vi "HMI.vi"(8 "error in (no error)":errorcluster caption="entrée d'erreur (pas d'erreur)", 11 "Class Popup Autotest (Default) en entrée":refnum<class "Popup Autotest_Without_Actor.lvclass">) -> (0 "error out":errorcluster caption="sortie d'erreur", 1 "Input":string, 2 "Autotest":bool, 3 "Class Popup Autotest (Default) en sortie":refnum<class "Popup Autotest_Without_Actor.lvclass">)   [LabVIEW 2020, in "Library Instrument & Equipement.lvlib" / "Library Popup.lvlib" / "Popup Autotest_Without_Actor.lvclass"]
uses:
  Popup Autotest_Without_Actor.lvclass
  C:/Users/ngarcin/OneDrive - Altyor/Standard TB/Class/Popup/Class Popup (Main)/Class Popup (Main).lvclass
  C:/Users/ngarcin/OneDrive - Altyor/Standard TB/Class/Popup/Class Popup Autotest (Default)/Popup Autotest (Default).lvclass
  Commun VI/TypeDef/Commande Popup autotest/Commande element autotest.ctl
  Variable Instr.vi
  Instrument/Instrument (Default)/Class Instrument (Default).lvclass
  Class Popup Autotest (Default)/Popup Autotest (Default).lvclass
  Popup Autotest_Without_Actor.lvclass/Popup Autotest_Without_Actor.ctl
panel:
  out "Element test":T2
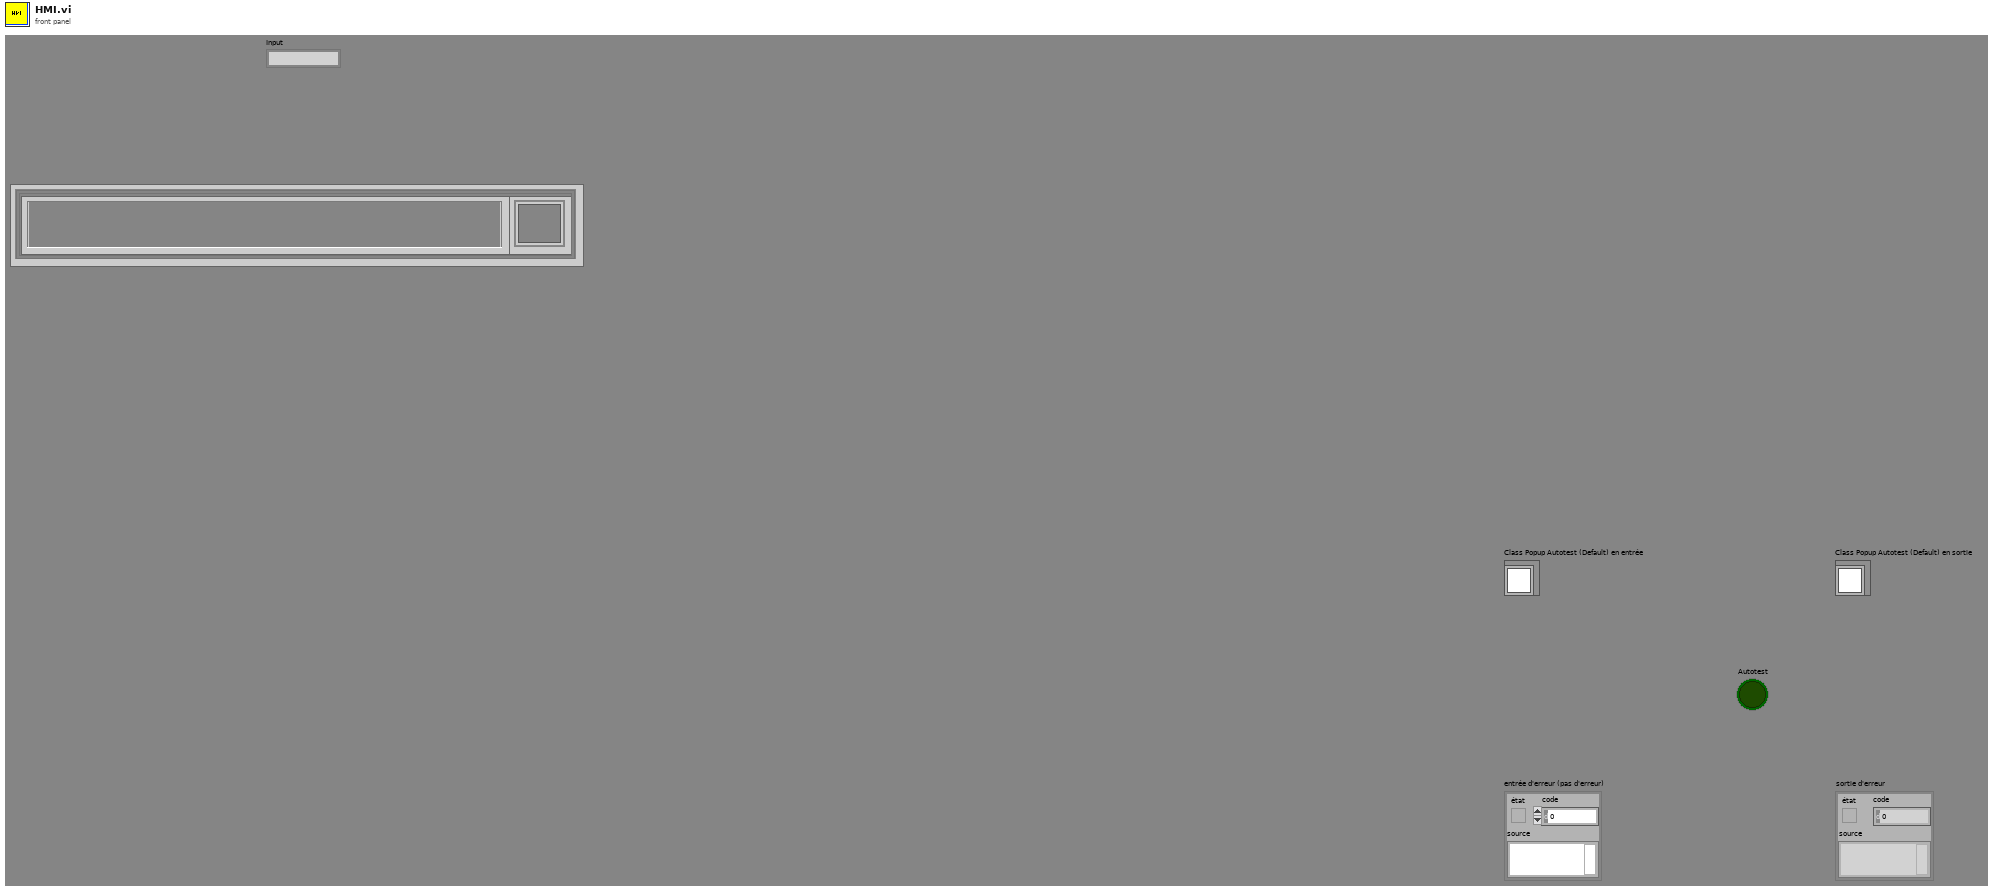
[diagram p1: front panel]
types:
  T1 = typedef "Commande element autotest.ctl" = cluster{"Instrument":string, "Etat":cluster{"Menu déroulant":u16}}
  T2 = cluster{"Element autotest":T1, "Element autotest 2":T1, "Element autotest 3":T1, "Element autotest 4":T1, "Element autotest 5":T1, "Element autotest 6":T1, "Element autotest 7":T1, "Element autotest 8":T1, "Element autotest 9":T1}
  T3 = cluster{"Name":string, "Instrument":refnum<class "Class Instrument (Default).lvclass">, "Close After Autotest":bool}[]
  T4 = cluster{"Name":string, "Instrument":refnum<class "Class Instrument (Default).lvclass">, "Close After Autotest":bool}
  T5 = typedef "LVRectTypeDef.ctl" = cluster{"Left":i16, "Top":i16, "Right":i16, "Bottom":i16}
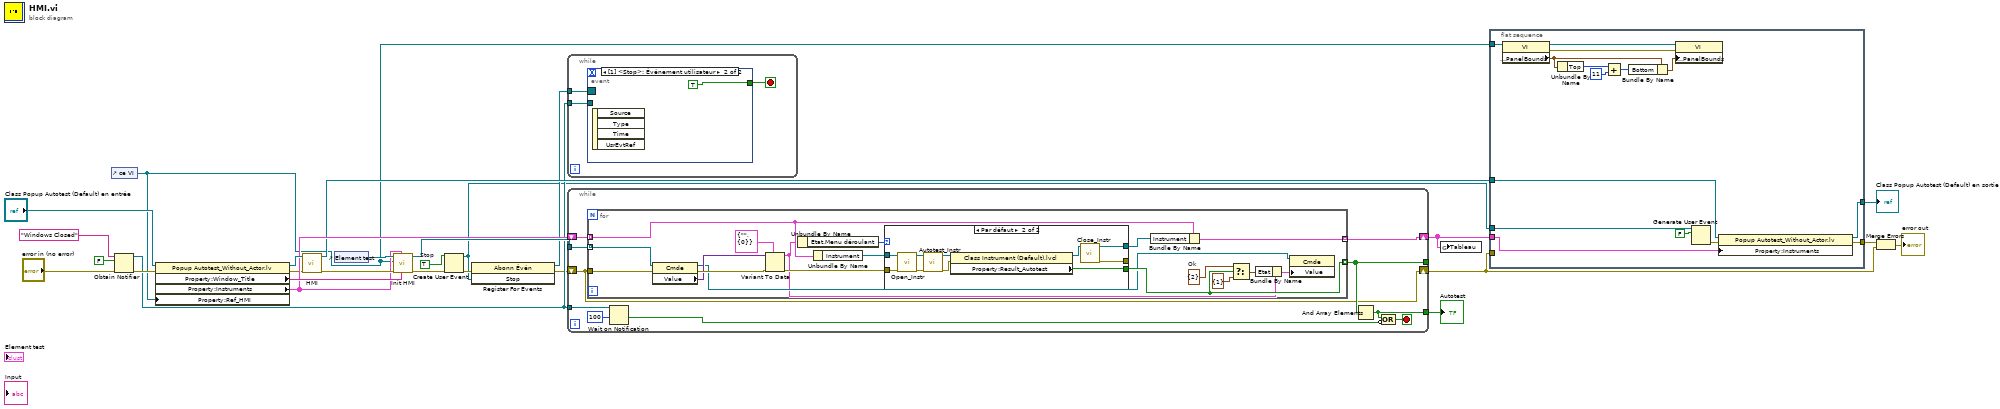
[diagram p0: block diagram]
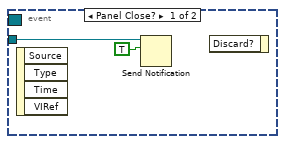
[diagram p2: hidden frame]
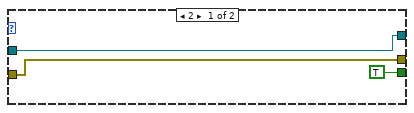
[diagram p3: hidden frame]
diagram:
  w12 = TRUE  # Stop
  n1 = control-ref of="ce VI"() -> (w1:refnum<vi>)
  n2 = Obtain Notifier(name (unnamed)="Windows Closed" ("nom (aucun)"), notification data type=FALSE, error in (no error)="error in (no error)") -> (notifier out=w14:refnum<notifier>, error out=w17:errorcluster)  [unwired: 1 in, 1 out]
  n3 = property class="Popup Autotest_Without_Actor.lv"(reference="Class Popup Autotest (Default) en entrée", error in=w17, "Property:Ref_HMI"=w1) -> (reference out=w27:refnum<class "Popup Autotest_Without_Actor.lvclass">, error out=w2:errorcluster, "Property:Window_Title"=w24:string, "Property:Instruments"=w21:T3)
  n4 = call-parent "HMI.vi"("error in (no error)"=w2, "Class Popup Autotest (Default) en entrée"=w27) -> ("error out"=w23:errorcluster, "Class Popup Autotest (Default) en sortie"=w18:refnum<class "Popup Autotest_Without_Actor.lvclass">)  [unwired: 6 in, 2 out]
  n5 = control-ref of="Element test"() -> (w25:refnum<vi>)
  n6 = call "Init HMI.vi"("Window_Title"=w24, "Instruments"=w21, "entrée d'erreur (pas d'erreur)"=w23, "ce VI"=w1, "Cluster en entrée"=w25) -> ("sortie d'erreur"=w11:errorcluster, "Ref Cmd Cluster element"=w22:refnum<vi>[])  [unwired: 5 in]
  n7 = Create User Event(user event datatype=w12, error in=w11) -> (user event=w8:refnum<user-event>, error out=w10:errorcluster)
  n8 = register-events(error in=w10, w8) -> (reference out=w13:refnum<event-registration>, error out=w9:errorcluster)  [unwired: 1 in]
  n9 = while {
    tunnel: w14 -> [w30]
    tunnel: w13 -> [w29]
    stop <- w28 stop-if-true
    n10 = event shown="[1] <Stop>: Événement utilisateur" {
      selector: w29 -> [_ _]
      dyn-events: _ -> [_ _]
      timeout: _ -> [_ _]
      tunnel: w30 -> [w32 _]
      tunnel: [_ TRUE] -> w28
      event Panel Close? {
        n11 = event-data() -> ()  [unwired: 1 in, 4 out]
        n12 = Send Notification(notification=TRUE, notifier=w32) -> ()  [unwired: 1 in, 2 out]
        n13 = event-data() -> ()  [unwired: 2 in, 1 out]
      }
      event User Event {
        n14 = event-data() -> ()  [unwired: 1 in, 4 out]
      }
    }
  }
  n15 = while {
    tunnel: [w38] -> _
    tunnel: w22 -> [w43]
    shift-right: [w34] -> w4
    shift-left: w9 -> [w34]
    shift-right: [w41] -> w3
    shift-left: w21 -> [w42]
    tunnel: w14 -> [w40]
    tunnel: [w37] -> w7
    stop <- w35 stop-if-true
    n16 = for {
      tunnel: w42 -> [w61] mode=indexing
      tunnel: [w60] -> w41 mode=indexing
      tunnel: [w55] -> w38 mode=indexing
      tunnel: w43 -> [w57] mode=indexing
      tunnel: w34 -> [w44]
      w56 = cluster{"Menu déroulant":u16} {"Menu déroulant"=2}  # Ok
      n17 = property class="Cmde"(reference=w57, error in=w44) -> (reference out=w51:refnum<vi>, error out=w58:errorcluster, "Value"=w53:variant)
      n18 = Variant To Data(error in=w58, type=T1 {"Instrument"="", "Etat"={"Menu déroulant"=0}} ("Element autotest"), Variant=w53) -> (data=w46:T1, error out=w48:errorcluster)
      n19 = Unbundle By Name(w46) -> ("Etat.Menu déroulant"=w45:u16)
      n20 = Unbundle By Name(w61) -> ("Instrument"=w47:refnum<class "Class Instrument (Default).lvclass">)
      n21 = case shown="Par défaut" w45 {
        tunnel: [w64 w66] -> w59
        tunnel: [TRUE ("Property:Result_Autotest") w72] -> w55
        tunnel: [w63 w65] -> _
        tunnel: w48 -> [w63 w71]
        tunnel: w47 -> [w64 w69]
        frame 2 {
        }
        frame Default {
          n22 = call-dynamic "Open_Instr.vi"("error in (no error)"=w71, "Class Multimeter (Default) en entrée"=w69) -> ("error out"=w70:errorcluster, "Class Multimeter (Default) en sortie"=w68:refnum<class "Class Instrument (Default).lvclass">)  [unwired: 8 in]
          n23 = call-dynamic "Autotest_Instr.vi"("error in (no error)"=w70, "Class Instrument (Default) en entrée"=w68) -> ("error out"=w73:errorcluster, "Class Instrument (Default) en sortie"=w74:refnum<class "Class Instrument (Default).lvclass">)  [unwired: 8 in]
          n24 = property class="Class Instrument (Default).lvcl"(reference=w74, error in=w73) -> (reference out=w67:refnum<class "Class Instrument (Default).lvclass">, "Property:Result_Autotest"=w72:bool)  [unwired: 1 out]
          n25 = call-dynamic "Close_Instr.vi"("Class Instrument (Default) en entrée"=w67) -> ("error out"=w65:errorcluster, "Class Instrument (Default) en sortie"=w66:refnum<class "Class Instrument (Default).lvclass">)  [unwired: 9 in]
        }
      }
      n26 = Bundle By Name(cluster=w61, "Instrument"=w59) -> (w60:T4)
      n27 = Select(t=w56, s=w55, f=cluster{"Menu déroulant":u16} {"Menu déroulant"=1} ("cas faux")) -> (s? t:f=w49:cluster{"Menu déroulant":u16})
      n28 = Bundle By Name(cluster=w46, "Etat"=w49) -> (w50:T1)
      n29 = property class="Cmde"(reference=w51, "Value"=w50) -> ()  [unwired: 1 in, 2 out]
    }
    n30 = Wait on Notification(notifier=w40, timeout in ms (-1)=100 ("timeout en ms (-1)")) -> (timed out?=w36:bool)  [unwired: 2 in, 3 out]
    n31 = And Array Elements(Boolean array=w38) -> (logical AND=w37:bool)
    n32 = Compound Arithmetic op=OR ("Opérateur arithmétique")(w37, invert w36) -> (w35:bool)
  }
  "Autotest" <- w7
  n33 = global write "Variable Instr.vi" "Tableau"(w3) -> ()
  n34 = flat-sequence {
    tunnel: [w89] -> w20
    tunnel: w18 -> [w88]
    tunnel: w3 -> [w87]
    tunnel: w8 -> [w85]
    tunnel: [w83] -> w6
    tunnel: w4 -> [_]
    tunnel: w1 -> [w75]
    frame #0 {
      n35 = property class="VI"(reference=w75) -> (reference out=w80:refnum<vi>, error out=w82:errorcluster, "Front Panel.PanelBounds"=w81:T5)  [unwired: 1 in]
      n36 = Unbundle By Name(w81) -> ("Top"=w79:i16)
      n37 = Add(x=w79, y=i16 11) -> (x+y=w78:i16)
      n38 = Bundle By Name(cluster=w81, "Bottom"=w78) -> (w77:T5)
      n39 = property class="VI"(reference=w80, error in=w82, "Front Panel.PanelBounds"=w77) -> ()  [unwired: 2 out]
      n40 = Generate User Event(user event=w85, event data cluster=FALSE ("données d'événement")) -> (error out=w86:errorcluster)  [unwired: 2 in, 1 out]
      n41 = property class="Popup Autotest_Without_Actor.lv"(reference=w88, error in=w86, "Property:Instruments"=w87) -> (reference out=w89:refnum<class "Popup Autotest_Without_Actor.lvclass">, error out=w83:errorcluster)
    }
  }
  n42 = Merge Errors(w6, w4) -> (→"error out":errorcluster)
  "Class Popup Autotest (Default) en sortie" <- w20
